vi "MoveOut.vi"(8 "error in (no error)":errorcluster, 10 "Destination":string, 11 "reference in":refnum<class "DUT_Handler_Simple.lvclass">) -> (0 "error out":errorcluster, 3 "reference in":refnum<class "DUT_Handler_Simple.lvclass">)   [LabVIEW 2022 SP3, in "DUT_Handler_Simple.lvlib" / "DUT_Handler_Simple.lvclass"]
uses:
  DUT_Handler_Simple.lvclass
  Components/DUT_Handler_Base.lvlibp/Action.ctl
  Components/DUT_Handler_Base.lvlibp/DUT_Handler_Base.lvclass
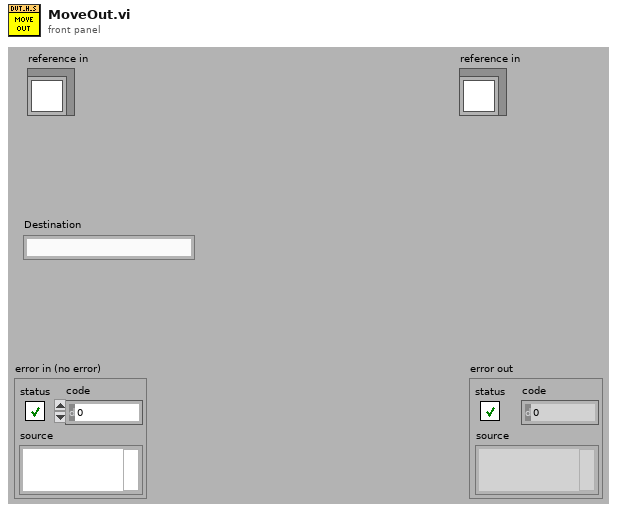
[diagram p1: front panel]
types:
  T1 = typedef "DUT_Handler_Base.lvlibp/DUT_Handler_Base.lvclass/Action.ctl" = enum16{"Load", "Cancel", "MoveIn", "MoveOut", "Abort", "Msg", "Enabled", "Disabled", "Fault", "Shutdown"}
  T2 = typedef "DUT_Handler_Simple.lvlib/DUT_Handler_Simple.lvclass/ObjectAttributes.ctl" = cluster{"Config":T3, "event_data":T4, "Enabled":bool, "Barcode_Reader":refnum<class "Barcode_Reader_Base.lvclass">}
  T3 = typedef "DUT_Handler_Simple.lvlib/DUT_Handler_Simple.lvclass/Config.ctl" = cluster{"default":string}
  T4 = typedef "DUT_Handler_Base.lvlibp/DUT_Handler_Base.lvclass/EventData.ctl" = cluster{"Action":enum16{"Load", "Cancel", "MoveIn", "MoveOut", "Abort", "Msg", "Enabled", "Disabled", "Fault", "Shutdown"}, "SN":string, "BN":string, "DUT__ID":u32, "Message":string, "From":string, "To":string}
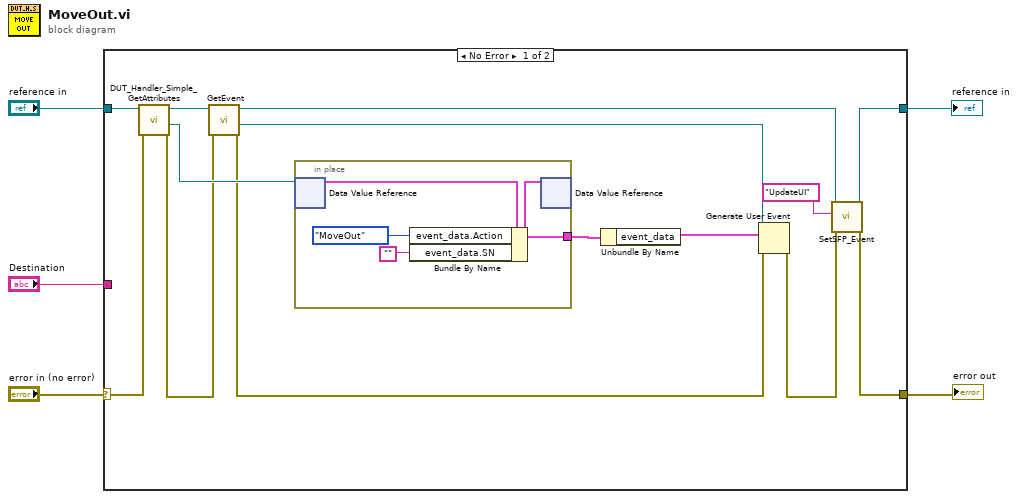
[diagram p0: block diagram]
diagram:
  n1 = case shown="No Error" "error in (no error)" {
    selector: "error in (no error)" -> [w19 w25]
    tunnel: [w11 w25] -> w4
    tunnel: [w13 w24] -> w2
    tunnel: "reference in" -> [w18 w24]
    tunnel: "Destination" -> [_ _]
    frame No Error {
      n2 = call "DUT_Handler_Simple_GetAttributes.vi"("error in (no error)"=w19, "reference in"=w18) -> ("error out"=w15:errorcluster, "DataRef"=w17:refnum<data-value>, "reference out"=w16:refnum<class "DUT_Handler_Simple.lvclass">)  [unwired: 6 in, 1 out]
      n3 = call-dynamic "GetEvent.vi"("error in (no error)"=w15, "reference in"=w16) -> ("error out"=w9:errorcluster, "DUT_Handler"=w8:refnum<user-event>, "reference in"=w12:refnum<class "DUT_Handler_Simple.lvclass">)  [unwired: 6 in]
      n4 = in-place {
        in-place-border: [w22] -> w7
        n5 = in-place-dvr #1(w17) -> (w23:T2)  [unwired: 1 out]
        n6 = Bundle By Name(cluster=w23, "event_data.Action"=Action."MoveOut" ("Action"), "event_data.SN"="") -> (w22:T2)
        n7 = in-place-dvr #1(w22) -> ()  [unwired: 2 out]
      }
      n8 = Unbundle By Name(w7) -> ("event_data"=w6:T4)
      n9 = Generate User Event(user event=w8, event data cluster=w6, error in=w9) -> (error out=w10:errorcluster)  [unwired: 1 in, 1 out]
      n10 = call-dynamic "SetSFP_Event.vi"("error in (no error)"=w10, "msg"="UpdateUI", "reference in"=w12) -> ("error out"=w11:errorcluster, "reference out"=w13:refnum<class "DUT_Handler_Simple.lvclass">)  [unwired: 7 in]
    }
    frame Error {
    }
  }
  "error out" <- w4
  "reference in" <- w2
